vi "Insight_Measure_DataStreaming_Enable.vi"(8 "error in (no error)":errorcluster, 9 "Mode (Read / Write)":enum8{"Write", "Read"}(ring), 10 "Data Streaming (Off)":enum16{"Off", "On"}(ring), 11 "telnet connection":T1) -> (0 "error out":errorcluster, 1 "Data Streaming":enum16{"Off", "On"}(ring), 2 "response data":string, 3 "telnet  connection out":T1)   [LabVIEW 2011]
doc: "Insight Photonic Solutions\n\nThis VI enables or disables Data Streaming when the laser is in Measurement Mode.\n\nver 1.0 - original release"
uses:
  Telnet Session.ctl
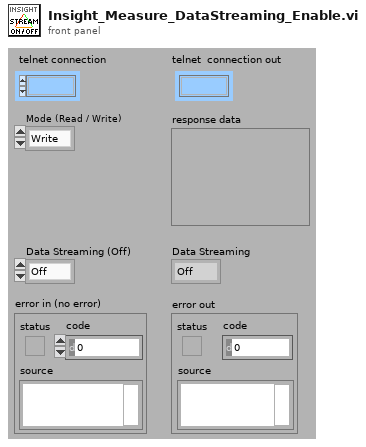
[diagram p1: front panel]
types:
  T1 = typedef "Telnet Session.ctl" = refnum<k1>
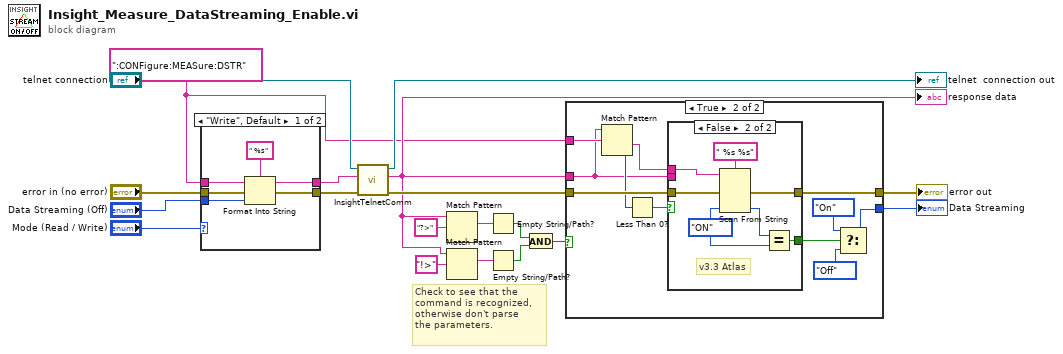
[diagram p0: block diagram]
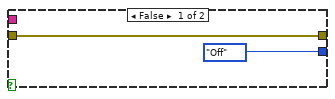
[diagram p2: hidden frame]
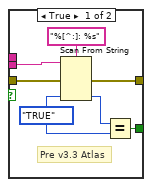
[diagram p3: hidden frame]
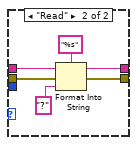
[diagram p4: hidden frame]
diagram:
  w1 = ":CONFigure:MEASure:DSTR" ("String")
  # "Check to see that the \ncommand is recognized,\notherwise don't parse \nthe parameters."
  n1 = case shown="\"Write\", Default" "Mode (Read / Write)" {
    tunnel: [w25 w27] -> w16
    tunnel: "error in (no error)" -> [w24 w26]
    tunnel: w1 -> [w23 w29]
    tunnel: "Data Streaming (Off)" -> [w22 _]
    tunnel: [w20 w28] -> w14
    frame "Write", Default {
      n2 = Format Into String(format string=" %s", initial string=w23, error in=w24, w22) -> (resulting string=w20:string, error out=w25:errorcluster)
    }
    frame "Read" {
      n3 = Format Into String(format string="%s", initial string=w29, error in=w26, "?" ("input 1")) -> (resulting string=w28:string, error out=w27:errorcluster)
    }
  }
  n4 = call "InsightTelnetComm.vi"("error in"=w16, "write buffer (\"\")"=w14, "telnet connection"="telnet connection") -> ("error out"=w15:errorcluster, "response data"=w3:string, "telnet  connection out"=→"telnet  connection out":T1)  [unwired: 4 in]
  "response data" <- w3
  n5 = Match Pattern(string=w3, regular expression="?>") -> (match substring=w8:string)  [unwired: 1 in, 3 out]
  n6 = Match Pattern(string=w3, regular expression="!>") -> (match substring=w7:string)  [unwired: 1 in, 3 out]
  n7 = Empty String/Path?(string/path=w8) -> (empty?=w5:bool)
  n8 = Empty String/Path?(string/path=w7) -> (empty?=w4:bool)
  n9 = And(x=w5, y=w4) -> (x .and. y?=w2:bool)
  n10 = case shown="True" w2 {
    tunnel: [w33 w44] -> w17
    tunnel: w15 -> [w33 w43]
    tunnel: [enum16{"Off", "On"}."Off" ("Data Streaming (Off)") w41] -> w10
    tunnel: w3 -> [_ w35]
    tunnel: w1 -> [_ w36]
    frame False {
    }
    frame True {
      n11 = Match Pattern(string=w35, regular expression=w36) -> (after substring=w34:string, offset past match=w38:i32)  [unwired: 1 in, 2 out]
      n12 = Less Than 0?(x=w38) -> (x < 0?=w37:bool)
      n13 = case shown="False" w37 {
        tunnel: [w50 w57] -> w44
        tunnel: w43 -> [w49 w56]
        tunnel: w35 -> [w48 _]
        tunnel: [w47 w55] -> w42
        tunnel: w34 -> [_ w52]
        frame True {
          w45 = enum16{"FALSE", "TRUE"}."TRUE" ("Data Streaming")
          # "Pre v3.3 Atlas"
          n14 = Scan From String(format string="%[^:]: %s", input string=w48, error in=w49, default 2=w45) -> (error out=w50:errorcluster, output 2=w46:enum16{"FALSE", "TRUE"})  [unwired: 3 in, 2 out]
          n15 = Equal?(x=w46, y=w45) -> (x = y?=w47:bool)
        }
        frame False {
          w53 = enum16{"ON", "OFF"}."ON" ("Data Streaming")
          # "v3.3 Atlas"
          n16 = Scan From String(format string=" %s %s", input string=w52, error in=w56, default 2=w53) -> (error out=w57:errorcluster, output 2=w54:enum16{"ON", "OFF"})  [unwired: 3 in, 2 out]
          n17 = Equal?(x=w54, y=w53) -> (x = y?=w55:bool)
        }
      }
      n18 = Select(t=enum16{"Off", "On"}."On" ("Data Streaming (Off)"), s=w42, f=enum16{"Off", "On"}."Off" ("Data Streaming (Off)")) -> (s? t:f=w41:enum16{"Off", "On"})
    }
  }
  "error out" <- w17
  "Data Streaming" <- w10
